vi "getValuesArray.vi"(8 "error in":errorcluster, 9 "timeout in ms (-1)":i32=100, 11 "appended array":refnum<notifier>[](array[refnum])) -> (0 "error out":errorcluster, 2 "notifier values":string[](array[string]), 3 "notifier names":string[](array[string]))   [LabVIEW 2013]
doc: "Takes an array of notifiers and returns two arrays containing the name and value of each notifier. All values have been flattened to strings.\nNotifier value must be a 1d array of doubles.\n\nKaitlin Gallagher\n3/4/14"
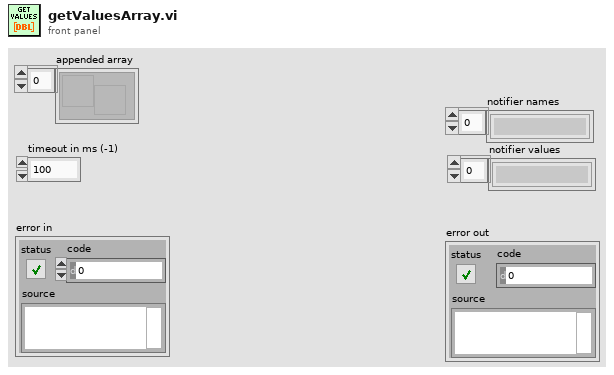
[diagram p1: front panel]
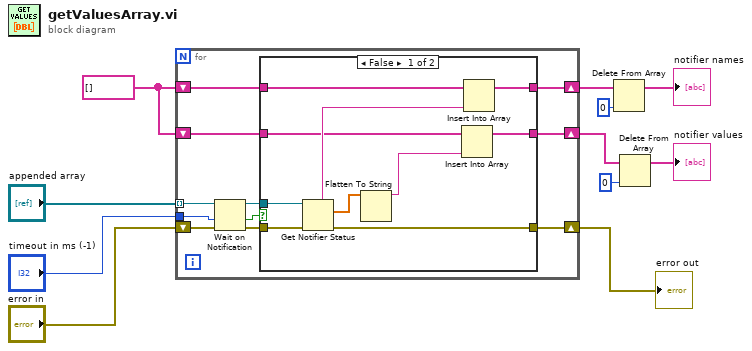
[diagram p0: block diagram]
diagram:
  w2 = string[] [] ("notifier names 2")
  n1 = for {
    shift-right: [w22] -> w10
    shift-left: "error in" -> [w20]
    tunnel: "timeout in ms (-1)" -> [w18]
    shift-right: [w15] -> w8
    shift-left: w2 -> [w16]
    shift-right: [w13] -> w5
    shift-left: w2 -> [w14]
    tunnel: "appended array" -> [w12] mode=indexing
    n2 = Wait on Notification(notifier=w12, timeout in ms (-1)=w18, error in (no error)=w20) -> (notifier out=w21:refnum<notifier>, timed out?=w17:bool, error out=w19:errorcluster)  [unwired: 1 in, 1 out]
    n3 = case shown="False" w17 {
      tunnel: [w32 w35] -> w22
      tunnel: w21 -> [w30 _]
      tunnel: w19 -> [w29 w35]
      tunnel: w16 -> [w28 w34]
      tunnel: [w27 w34] -> w15
      tunnel: w14 -> [w24 w33]
      tunnel: [w23 w33] -> w13
      frame False {
        n4 = Get Notifier Status(notifier=w30, error in (no error)=w29) -> (notifier name=w26:string, current notification=w31:dbl[], error out=w32:errorcluster)  [unwired: 2 out]
        n5 = Flatten To String(anything=w31) -> (data string=w25:string)  [unwired: 3 in, 2 out]
        n6 = Insert Into Array(array=w24, new element=w25) -> (w23:string[])  [unwired: 1 in]
        n7 = Insert Into Array(array=w28, new element=w26) -> (w27:string[])  [unwired: 1 in]
      }
      frame True {
      }
    }
  }
  "error out" <- w10
  n8 = Delete From Array(array=w8, index=0) -> (array with subset deleted=→"notifier names":string[])  [unwired: 1 in, 1 out]
  n9 = Delete From Array(array=w5, index=0) -> (array with subset deleted=→"notifier values":string[])  [unwired: 1 in, 1 out]
